vi "Add Sections and Channels.vi"(8 "error in (no error)":errorcluster, 11 "Device Item Ref in":T1 format="%.0x") -> (0 "error out":errorcluster, 3 "Item Ref out":T1 format="%.0x")   [LabVIEW 2020, in "PXI-2510 System Explorer.lvlib"]
uses:
  PXI-2510 System Explorer.lvlib
  <vilib>/NI VeriStand/Custom Device API/Custom Device Item Ref.ctl
  <vilib>/NI VeriStand/Custom Device API/Custom Device Channel Type.ctl
  <vilib>/NI VeriStand/Custom Device API/Custom Device Channel.ctl
  Types/Fault Bus Input Selector.ctl
  Shared/Constants.vi
  <vilib>/NI VeriStand/Custom Device API/Set Item Property (String).vi
  <vilib>/NI VeriStand/Custom Device API/Custom Device API.lvlib
  Shared/PXI-2510 Shared.lvlib
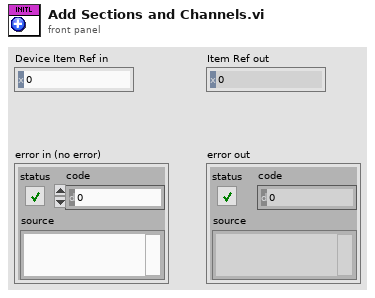
[diagram p1: front panel]
types:
  T1 = typedef "Custom Device API.lvlib/Custom Device Item Ref.ctl" = u64
  T2 = typedef "Custom Device API.lvlib/Custom Device Channel Type.ctl" = enum16{"Input", "Output"}
  T3 = typedef "Custom Device API.lvlib/Custom Device Channel.ctl" = cluster{"Type":T2, "Units":string, "Default Value":dbl, "Faultable":bool, "Scalable":bool}
  T4 = typedef "PXI-2510 System Explorer.lvlib/Fault Bus Input Selector.ctl" = enum16{"Default", "Input 0", "Input 1", "Input 2", "Input 3", "Main Bus Only"}
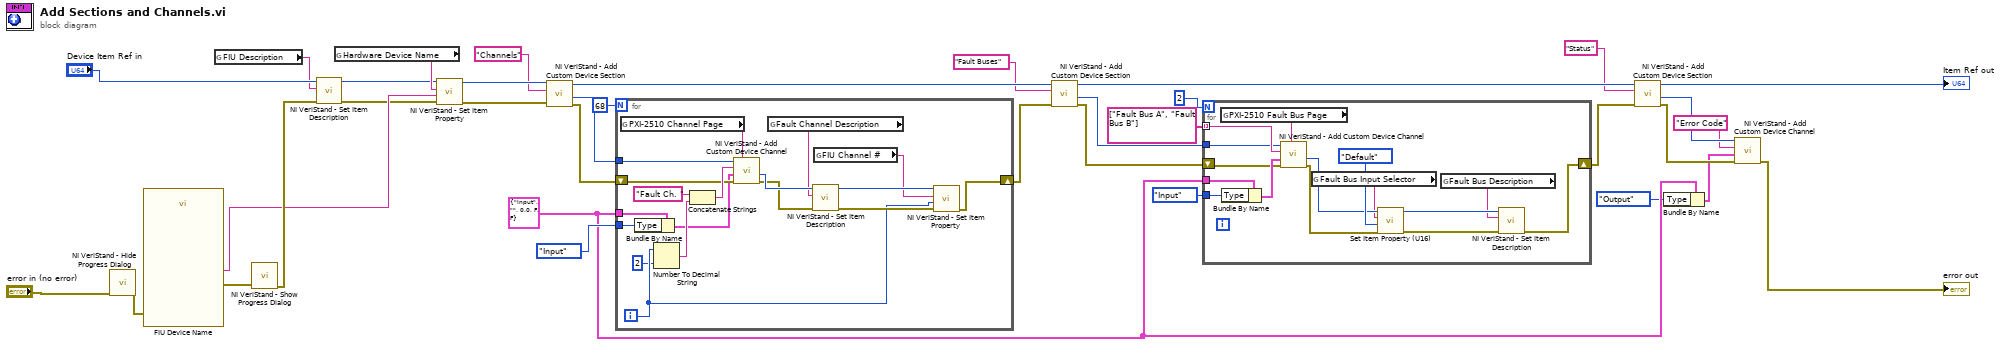
[diagram p0: block diagram]
diagram:
  w5 = T3 {"Type"=enum."Input", "Units"="", "Default Value"=0.0, "Faultable"=FALSE, "Scalable"=FALSE} ("Channel")
  n1 = call <vilib>:"NI VeriStand - Hide Progress Dialog.vi"("error in (no error)"="error in (no error)") -> ("error out"=w36:errorcluster)  [unwired: 10 in]
  n2 = call "FIU Device Name"("error in (no error)"=w36) -> ("MAX Device Name"=w30:string, "error out"=w34:errorcluster)  [unwired: 16 in, 1 out]
  n3 = global read "Constants.vi" "FIU Description"() -> (w31:string)
  n4 = call <vilib>:"NI VeriStand - Show Progress Dialog.vi"("error in (no error)"=w34) -> ("error out"=w33:errorcluster)  [unwired: 10 in]
  n5 = call <vilib>:"NI VeriStand - Set Item Description.vi"("error in (no error)"=w33, "Description"=w31, "Item Ref in"="Device Item Ref in") -> ("error out"=w27:errorcluster, "Item Ref out"=w28:T1)  [unwired: 6 in, 1 out]
  n6 = global read "Constants.vi" "Hardware Device Name"() -> (w29:string)
  n7 = call-poly <vilib>:"NI VeriStand - Set Item Property.vi"("error in (no error)"=w27, "Value"=w30, "Property Name"=w29, "Item Ref in"=w28) -> ("error out"=w25:errorcluster, "Item Ref out"=w26:T1)  [unwired: 5 in, 1 out]
  n8 = call <vilib>:"NI VeriStand - Add Custom Device Section.vi"("error in (no error)"=w25, "Section Name"="Channels", "Parent Ref in"=w26) -> ("error out"=w22:errorcluster, "Section Ptr"=w23:T1, "Parent Ref out"=w21:T1)  [unwired: 5 in, 1 out]
  n9 = for {
    N: 68 -> [_]
    tunnel: w23 -> [w54]
    shift-right: [w42] -> w20
    shift-left: w22 -> [w50]
    tunnel: w5 -> [w40]
    tunnel: Custom_Device_Channel_Type."Input" ("Type") -> [w39]
    i -> [w43]
    n10 = global read "Constants.vi" "PXI-2510 Channel Page"() -> (w37:string)
    n11 = Bundle By Name(cluster=w40, "Type"=w39) -> (w38:T3)
    n12 = Number To Decimal String(number=w43, width (-)=i16 2) -> (decimal integer string=w51:string)
    n13 = Concatenate Strings("Fault Ch. " ("string"), w51) -> (w53:string)
    n14 = call <vilib>:"NI VeriStand - Add Custom Device Channel.vi"("GUID (Default Channel)"=w37, "error in (no error)"=w50, "Channel"=w38, "Channel Name"=w53, "Parent Ref in"=w54) -> ("error out"=w48:errorcluster, "Channel Ref"=w49:T1)  [unwired: 3 in, 2 out]
    n15 = global read "Constants.vi" "Fault Channel Description"() -> (w47:string)
    n16 = call <vilib>:"NI VeriStand - Set Item Description.vi"("error in (no error)"=w48, "Description"=w47, "Item Ref in"=w49) -> ("error out"=w45:errorcluster, "Item Ref out"=w46:T1)  [unwired: 6 in, 1 out]
    n17 = global read "Constants.vi" "FIU Channel #"() -> (w44:string)
    n18 = call-poly <vilib>:"NI VeriStand - Set Item Property.vi"("error in (no error)"=w45, "Value"=w43, "Property Name"=w44, "Item Ref in"=w46) -> ("error out"=w42:errorcluster)  [unwired: 5 in, 2 out]
  }
  n19 = call <vilib>:"NI VeriStand - Add Custom Device Section.vi"("error in (no error)"=w20, "Section Name"="Fault Buses", "Parent Ref in"=w21) -> ("error out"=w15:errorcluster, "Section Ptr"=w16:T1, "Parent Ref out"=w11:T1)  [unwired: 5 in, 1 out]
  n20 = for {
    N: 2 -> [_]
    tunnel: w5 -> [w69]
    tunnel: Custom_Device_Channel_Type."Input" ("Type") -> [w67]
    shift-right: [w58] -> w9
    shift-left: w15 -> [w66]
    tunnel: string[] ["Fault Bus A", "Fault Bus B"] -> [w64] mode=indexing
    tunnel: w16 -> [w62]
    n21 = global read "Constants.vi" "PXI-2510 Fault Bus Page"() -> (w55:string)
    n22 = Bundle By Name(cluster=w69, "Type"=w67) -> (w68:T3)
    n23 = call <vilib>:"NI VeriStand - Add Custom Device Channel.vi"("GUID (Default Channel)"=w55, "error in (no error)"=w66, "Channel"=w68, "Channel Name"=w64, "Parent Ref in"=w62) -> ("error out"=w65:errorcluster, "Channel Ref"=w61:T1)  [unwired: 3 in, 2 out]
    n24 = global read "Constants.vi" "Fault Bus Input Selector"() -> (w57:string)
    n25 = call <vilib>:"Set Item Property (U16).vi"("error in (no error)"=w65, "Value"=Fault_Bus_Input_Selector."Default" ("Fault Bus Input Selector"), "Property Name"=w57, "Item Ref in"=w61) -> ("error out"=w59:errorcluster, "Item Ref out"=w60:T1)  [unwired: 5 in, 1 out]
    n26 = global read "Constants.vi" "Fault Bus Description"() -> (w56:string)
    n27 = call <vilib>:"NI VeriStand - Set Item Description.vi"("error in (no error)"=w59, "Description"=w56, "Item Ref in"=w60) -> ("error out"=w58:errorcluster)  [unwired: 6 in, 2 out]
  }
  n28 = call <vilib>:"NI VeriStand - Add Custom Device Section.vi"("error in (no error)"=w9, "Section Name"="Status", "Parent Ref in"=w11) -> ("error out"=w6:errorcluster, "Section Ptr"=w7:T1, "Parent Ref out"=→"Item Ref out":T1)  [unwired: 5 in, 1 out]
  n29 = Bundle By Name(cluster=w5, "Type"=Custom_Device_Channel_Type."Output") -> (w3:T3)
  n30 = call <vilib>:"NI VeriStand - Add Custom Device Channel.vi"("error in (no error)"=w6, "Channel"=w3, "Channel Name"="Error Code", "Parent Ref in"=w7) -> ("error out"=→"error out":errorcluster)  [unwired: 4 in, 3 out]
